vi "RoomNo.vi"(8 "error in (no error)":errorcluster, 10 "roomNumber":i32, 11 "Maze in":refnum<class "Maze.lvclass">) -> (0 "error out":errorcluster, 2 "Room*":refnum<data-value>, 3 "Maze out":refnum<class "Maze.lvclass">)   [LabVIEW 2016, in "Maze.lvclass"]
uses:
  Maze.lvclass
  Room/Room.lvclass
  Maze.lvclass/Maze.ctl
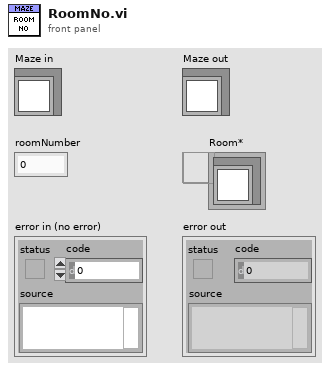
[diagram p1: front panel]
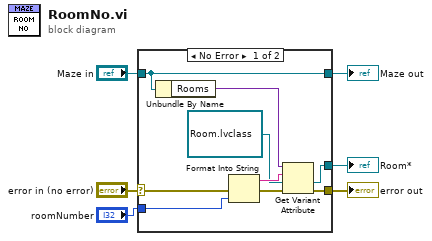
[diagram p0: block diagram]
diagram:
  n1 = case shown="No Error" "error in (no error)" {
    selector: "error in (no error)" -> [w9 w17]
    tunnel: [w7 w17] -> w5
    tunnel: [w15 w16] -> w3
    tunnel: "Maze in" -> [w15 w16]
    tunnel: "roomNumber" -> [w13 _]
    tunnel: [w10 _] -> w1
    frame No Error {
      n2 = Unbundle By Name(w15) -> ("Rooms"=w14:variant)
      n3 = Format Into String(error in=w9, w13) -> (resulting string=w12:string, error out=w8:errorcluster)  [unwired: 2 in]
      n4 = Get Variant Attribute(Variant=w14, name=w12, default value (empty Variant)=refnum<data-value> refnum ("Room*"), error in=w8) -> (value=w10:refnum<data-value>, error out=w7:errorcluster)  [unwired: 2 out]
    }
    frame Error {
    }
  }
  "error out" <- w5
  "Maze out" <- w3
  "Room*" <- w1
